vi "Receive Response.vi"(8 "error in (no error)":errorcluster, 9 "timeout in ms (0)":i32 format="%d ms", 11 "Plugin Thread in":refnum<class "Plugin Interface.lvclass">) -> (0 "error out":errorcluster, 2 "response":T1, 3 "Plugin Thread out":refnum<class "Plugin Interface.lvclass">)   [LabVIEW 2021, in "DSF Core.lvlib" / "Plugin Thread.lvclass"]
uses:
  Thread/Plugin/Plugin Thread.lvclass
  Interface/Plugin/Plugin Interface.lvclass
  Interface/Plugin/Response Data.ctl
  Interface/Plugin/Response.ctl
  Interface/Plugin/Response Parameters.ctl
  Interface/Plugin/Wait For Plugin Response.vi
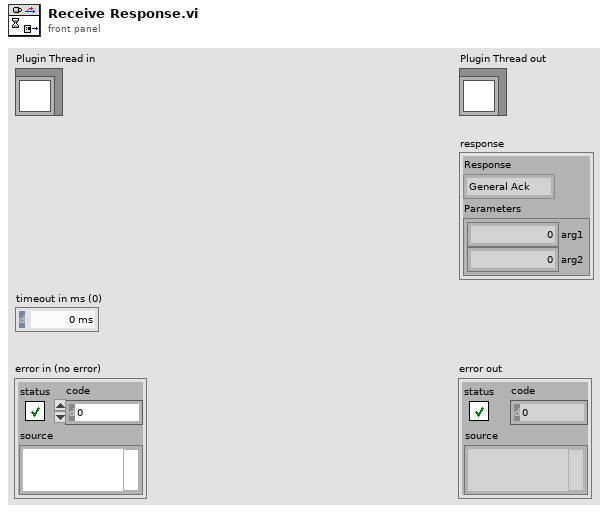
[diagram p1: front panel]
types:
  T1 = typedef "DSF Core.lvlib/Plugin Interface.lvclass/Response Data.ctl" = cluster{"Response":T2, "Parameters":T3}
  T2 = typedef "DSF Core.lvlib/Plugin Interface.lvclass/Response.ctl" = enum8{"General Ack", "Shutting Down"}
  T3 = typedef "DSF Core.lvlib/Plugin Interface.lvclass/Response Parameters.ctl" = cluster{"arg1":u64, "arg2":u64}
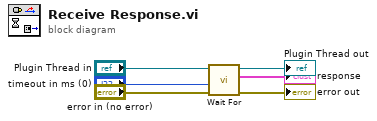
[diagram p0: block diagram]
diagram:
  n1 = call-poly "Wait For.vi"("error in (no error)"="error in (no error)", "timeout in ms (0)"="timeout in ms (0)", "Plugin Interface in"="Plugin Thread in") -> ("error out"=→"error out":errorcluster, "response"=→"response":T1, "Plugin Interface out"=→"Plugin Thread out":refnum<class "Plugin Interface.lvclass">)  [unwired: 5 in, 1 out]
